vi "SPD.Set Laser Power.vi"(8 "Error In":errorcluster, 10 "Pset":dbl, 11 "SPD.Stand Ctrl in":T1 {"spdDeviceSession"."hidSPD.Sturtup Values"."HV_bias" format="%#_6p, V"; "spdDeviceSession"."hidSPD.Sturtup Values"."TSet" format="%#_6p, DegC"; "spdDeviceSession"."hidSPD.Controller"."HV_bias" format="%#_6p, V"; "spdDeviceSession"."hidSPD.Controller"."TSet" format="%#_6p, DegC"}) -> (0 "Error Out":errorcluster, 3 "SPD.Stand Ctrl out":T1 {"spdDeviceSession"."hidSPD.Sturtup Values"."HV_bias" format="%#_6p, V"; "spdDeviceSession"."hidSPD.Sturtup Values"."TSet" format="%#_6p, DegC"; "spdDeviceSession"."hidSPD.Controller"."HV_bias" format="%#_6p, V"; "spdDeviceSession"."hidSPD.Controller"."TSet" format="%#_6p, DegC"})   [LabVIEW 2018]
uses:
  typedefs/SPD.Stand Ctrl.ctl
  Instruments/SPD HID Interface/hidSPDLibForLabView/LibVIs/hidSPD Controls/hidSPD Device Session.ctl
  Instruments/SPD HID Interface/hidSPDLibForLabView/LibVIs/hidSPD Controls/hidSPD Controller.ctl
  Instruments/SPD HID Interface/hidSPDLibForLabView/LibVIs/hidSPD Controls/hidSPD SPD Type.ctl
  Instruments/KC705 DevBoard/typedefs/DevB.Session.ctl
  Instruments/KeySight 53230A/typedefs/FreqC.Session.ctl
  Instruments/KeySight 8164B/KeySight 8164B LAN InstrLib/typedefs/KeySight 8164B control.ctl
  Instruments/LeCroy SDA830/typedefs/LeCroy.Session.ctl
  typedefs/SPD.Events.ctl
  ConfigFile/SPD.Config File ctrl.ctl
  <vilib>/Utility/config.llb/Config Data RefNum.ctl
  typedefs/SPD.Meas Result.ctl
  typedefs/SPD.Queues.ctl
  typedefs/SPD.Stand state.ctl
  <vilib>/Utility/error.llb/Error Cluster From Error Code.vi
  <vilib>/ErrorRing/Error Ring.xnode
  Instruments/KeySight 8164B/KeySight 8164B LAN InstrLib.lvlib
  <vilib>/Utility/config.llb/NI_LVConfig.lvlib
  Instruments/SPD HID Interface/hidSPDLibForLabView/hidSPDLibForLabView.lvlib
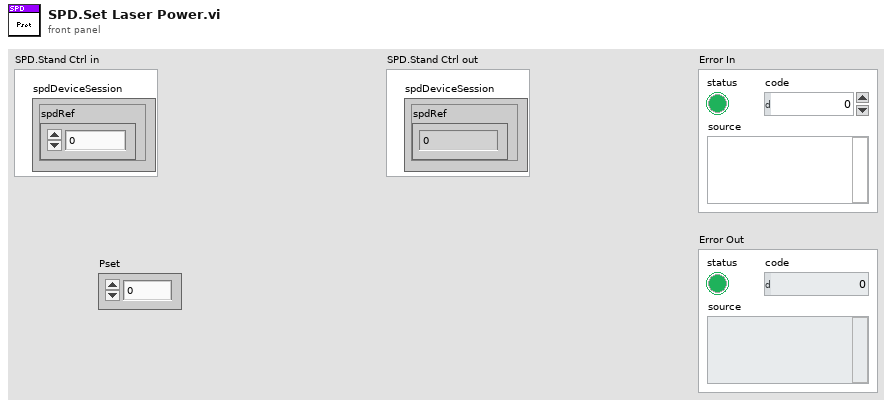
[diagram p1: front panel]
types:
  T1 = typedef "SPD.Stand Ctrl.ctl" = cluster{"spdDeviceSession":T2, "DevBSession":T5, "FreqCSession":T6, "8164BSession":T7, "LeCroySession":T8, "Events":T9, "configFile":T10, "SPD.Result":T12, "SPD.Queues":T13, "Console":refnum<vi>}
  T2 = typedef "hidSPDLibForLabView.lvlib/hidSPD Device Session.ctl" = cluster{"spdRef":u64, "connected":bool, "spdName":string, "hidSPD.Controller":T3, "hidSPD.Sturtup Values":T3, "SPD Type":T4}
  T3 = typedef "hidSPDLibForLabView.lvlib/hidSPD Controller.ctl" = cluster{"TSet":sgl, "HV_bias":sgl, "DDS_stb_code":u16}
  T4 = typedef "hidSPDLibForLabView.lvlib/hidSPD SPD Type.ctl" = enum16{"Free Run", "Gate"}
  T5 = typedef "DevB.Session.ctl" = cluster{"DevBRef":refnum<visa-resource-name>, "connected":bool}
  T6 = typedef "FreqC.Session.ctl" = cluster{"FreqCRef":refnum<visa-resource-name>, "timeout":dbl, "Gate":dbl, "connected":bool}
  T7 = typedef "KeySight 8164B LAN InstrLib.lvlib/KeySight 8164B control.ctl" = cluster{"Connection ID":refnum<k5>, "Connected":bool, "Info":string, "Slots Info":string[]}
  T8 = typedef "LeCroy.Session.ctl" = cluster{"LeCroySession":refnum<visa-resource-name>, "connected":bool}
  T9 = typedef "SPD.Events.ctl" = cluster{"DCRTest":refnum<user-event>, "Stop":refnum<user-event>}
  T10 = typedef "SPD.Config File ctrl.ctl" = cluster{"configFile ref":T11, "configFile path":path, "equipmentFile ref":T11}
  T11 = typedef "NI_LVConfig.lvlib/Config Data RefNum.ctl" = refnum<k1>
  T12 = typedef "SPD.Meas Result.ctl" = cluster{"HV_Bias":dbl[][][], "Stb_code":dbl[], "Temprature":dbl[], "Data":dbl[][][][], "DateTime":string}
  T13 = typedef "SPD.Queues.ctl" = cluster{"state queue":refnum<queue>}
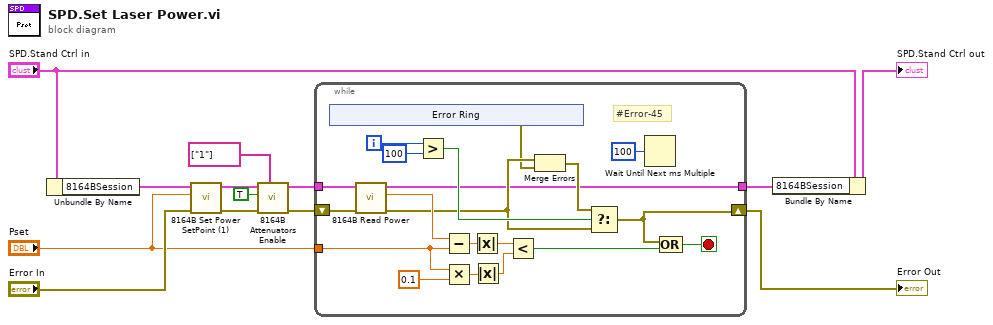
[diagram p0: block diagram]
diagram:
  n1 = Unbundle By Name("SPD.Stand Ctrl in") -> ("8164BSession"=w11:T7)
  n2 = call "8164B Set Power SetPoint (1).vi"("error in"="Error In", "Power Set Point"="Pset", "KeySight 8164B control in"=w11) -> ("error out"=w4:errorcluster, "KeySight 8164B control out"=w5:T7)  [unwired: 7 in]
  n3 = call "8164B Attenuators Enable.vi"("Slots"=string[] ["1"], "error in"=w4, "Enable"=TRUE, "KeySight 8164B control in"=w5) -> ("error out"=w2:errorcluster, "KeySight 8164B control out"=w3:T7)  [unwired: 6 in]
  n4 = while {
    tunnel: w3 -> [w33]
    shift-right: [w15] -> w9
    shift-left: w2 -> [w32]
    tunnel: "Pset" -> [w26]
    tunnel: [w14] -> w1
    i -> [w22]
    stop <- w16 stop-if-true
    # "#Error-45"
    n5 = xnode "Error Ring"() -> ("error out"=w17:errorcluster)
    n6 = call "8164B Read Power.vi"("error in"=w32, "KeySight 8164B control in"=w33) -> ("error out"=w18:errorcluster, "Power"=w25:dbl, "KeySight 8164B control out"=w14:T7)  [unwired: 7 in]
    n7 = Greater?(x=w22, y=100) -> (0:w20:bool)
    n8 = Subtract(x=w25, y=w26) -> (x-y=w31:dbl)
    n9 = Multiply(x=w26, y=0.1) -> (x*y=w29:dbl)
    n10 = Absolute Value(x=w31) -> (abs(x)=w28:dbl)
    n11 = Absolute Value(x=w29) -> (abs(x)=w27:dbl)
    n12 = Less?(x=w28, y=w27) -> (x < y?=w24:bool)
    n13 = Merge Errors(w18, w17) -> (w19:errorcluster)
    n14 = Select(t=w19, s=w20, f=w18) -> (s? t:f=w15:errorcluster)
    n15 = Wait Until Next ms Multiple(millisecond multiple=u32 100) -> ()  [unwired: 1 out]
    n16 = Compound Arithmetic op=OR(w15, w24) -> (w16:bool)
  }
  "Error Out" <- w9
  n17 = Bundle By Name(cluster="SPD.Stand Ctrl in", "8164BSession"=w1) -> (→"SPD.Stand Ctrl out":T1)
